vi "Thermistor_Callibration.vi"(11 "DataCluster in":T2={"Core"={"Current VI Reference"=refnum, "Close Panel on Exit?"=FALSE, "Exit"=FALSE, "Initialized?"=FALSE}, "Connections"={"cDAQ"={"Task"="", "Connected"=FALSE, "Active"=FALSE, "ID"=""}, "Camera"={"Session"="", "Connected"=FALSE, "Active"=FALSE, "Placeholder"=refnum}, "PSU"={"Port"="", "Connected"=FALSE, "Active"=FALSE}, "Arduino"={"Port"="", "Connected"=FALSE, "Active"=FALSE}}, "Data Acquisition"={"Setup"={"Label"="", "Operator"="", "Notes"="", "TempGrad"=1.0, "TargetTemp"=1.0, "Sample Volume"=1.0}, "Camera"={"Image"=refnum, "Save Image"=refnum, "Image Frequency"=20, "Rectangle"={"Left"=0, "Top"=0, "Right"=0, "Bottom"=0, "Rotation"=0.0}, "Calibration"={"Top Left"={"X"=0.0, "Y"=0.0}, "Top Right"={"X"=0.0, "Y"=0.0}, "Bottom Left"={"X"=0.0, "Y"=0.0}, "Bottom Right"={"X"=0.0, "Y"=0.0}, "Fixpoint"={"X"=0.0, "Y"=0.0}, "Scan Area"=0.0, "Fixpoint Area"=0.0, "Well Pixels"=[], "Valid"=FALSE}, "FocusPos"=0, "Display Mapping"=10}, "Thermistor"={"Sample Size"=1, "Calibration"={"B0.100"=[], "R25"=[], "c"=[], "State"=[], "V_S"=5.0, "R_S"=100.0}, "Timing Mode"=14713}, "Partition"={"Data"=[], "Cell Label"="", "Cell Color"=0, "Height"=10, "Width"=16, "Grid"=[]}, "Queue"={"Size"=1, "Queue"=refnum}, "Sample Rate"=1, "Active"=FALSE, "Ready"=FALSE, "Graph Mode"=0}, "Control"={"Sample Rate"=1, "PID gains"={"proportional gain (Kc)"=1.0, "integral time (Ti, min)"=0.01, "derivative time (Td, min)"=0.0}}} {"Control"."PID gains"."derivative time (Td, min)" format="%.3f"; "Control"."PID gains"."integral time (Ti, min)" format="%.3f"; "Control"."PID gains"."proportional gain (Kc)" format="%.3f"; "Control"."Sample Rate" min=1 max=20 step=1 format="%.0f Samples/sec"; "Data Acquisition"."Graph Mode" items=["Thermistor Temperature", "Camera Temperature"]; "Data Acquisition"."Thermistor"."Timing Mode" items=["Automatic"=16097, "High Resolution"=10195, "High Speed"=14712, "Best 50 Hz Rejection"=14713, "Best 60 Hz Rejection"=14714, "Custom"=10137]; "Data Acquisition"."Thermistor"."Calibration"."R_S" min=0.1 max=1000.0 format="%#_g kOhm"; "Data Acquisition"."Thermistor"."Calibration"."V_S" min=5.0 max=48.0 format="%#_g V"; "Data Acquisition"."Thermistor"."Calibration"."R25" min=0.1 max=1000.0 format="%#_g kOhm"; "Data Acquisition"."Thermistor"."Calibration"."B0.100" min=100.0 max=10000.0 format="%#_g K"; "Data Acquisition"."Thermistor"."Sample Size" min=1 max=200; "Data Acquisition"."Sample Rate" min=20 max=240 format="%.0f samples/min"; "Data Acquisition"."Queue"."Size" min=1 max=200; "Data Acquisition"."Camera"."Display Mapping" items=["Default"=10, "Most Significant Bits"=11, "Full Dynamic"=12, "Downshift"=13, "Given Range"=14, "90% Dynamic"=15, "Given Percent Range"=16]; "Data Acquisition"."Camera"."Calibration"."Fixpoint"."Y" format="%.2f"; "Data Acquisition"."Camera"."Calibration"."Fixpoint"."X" format="%.2f"; "Data Acquisition"."Camera"."Calibration"."Top Left"."Y" format="%.2f"; "Data Acquisition"."Camera"."Calibration"."Top Left"."X" format="%.2f"; "Data Acquisition"."Camera"."Calibration"."Top Right"."Y" format="%.2f"; "Data Acquisition"."Camera"."Calibration"."Top Right"."X" format="%.2f"; "Data Acquisition"."Camera"."Calibration"."Bottom Left"."Y" format="%.2f"; "Data Acquisition"."Camera"."Calibration"."Bottom Left"."X" format="%.2f"; "Data Acquisition"."Camera"."Calibration"."Bottom Right"."Y" format="%.2f"; "Data Acquisition"."Camera"."Calibration"."Bottom Right"."X" format="%.2f"; "Data Acquisition"."Camera"."Rectangle"."Rotation" min=-90.0 max=90.0 step=1.0 format="%.2f"; "Data Acquisition"."Camera"."Rectangle"."Left" scale=0.0..1024.0; "Data Acquisition"."Camera"."Rectangle"."Right" scale=0.0..1024.0; "Data Acquisition"."Camera"."Image Frequency" min=1 max=60 step=1; "Data Acquisition"."Setup"."Sample Volume" min=0.0 max=500.0 format="%#_g µL"; "Data Acquisition"."Setup"."TargetTemp" min=-40.0 max=40.0 step=0.5 format="%#_g °C"; "Data Acquisition"."Setup"."TempGrad" min=-100.0 max=100.0 step=0.1 format="%#_g °C/min"}) -> (2 "State Out":string="Data: Save Calibration", 3 "DataCluster out":T2={"Core"={"Current VI Reference"=refnum, "Close Panel on Exit?"=FALSE, "Exit"=FALSE, "Initialized?"=FALSE}, "Connections"={"cDAQ"={"Task"="", "Connected"=FALSE, "Active"=FALSE, "ID"=""}, "Camera"={"Session"="", "Connected"=FALSE, "Active"=FALSE, "Placeholder"=refnum}, "PSU"={"Port"="", "Connected"=FALSE, "Active"=FALSE}, "Arduino"={"Port"="", "Connected"=FALSE, "Active"=FALSE}}, "Data Acquisition"={"Setup"={"Label"="", "Operator"="", "Notes"="", "TempGrad"=0.0, "TargetTemp"=0.0, "Sample Volume"=0.0}, "Camera"={"Image"=refnum, "Save Image"=refnum, "Image Frequency"=20, "Rectangle"={"Left"=0, "Top"=0, "Right"=0, "Bottom"=0, "Rotation"=0.0}, "Calibration"={"Top Left"={"X"=0.0, "Y"=0.0}, "Top Right"={"X"=0.0, "Y"=0.0}, "Bottom Left"={"X"=0.0, "Y"=0.0}, "Bottom Right"={"X"=0.0, "Y"=0.0}, "Fixpoint"={"X"=0.0, "Y"=0.0}, "Scan Area"=0.0, "Fixpoint Area"=0.0, "Well Pixels"=[], "Valid"=FALSE}, "FocusPos"=0, "Display Mapping"=10}, "Thermistor"={"Sample Size"=0, "Calibration"={"B0.100"=[], "R25"=[], "c"=[], "State"=[], "V_S"=0.0, "R_S"=0.0}, "Timing Mode"=0}, "Partition"={"Data"=[], "Cell Label"="", "Cell Color"=0, "Height"=0, "Width"=0, "Grid"=[]}, "Queue"={"Size"=0, "Queue"=refnum}, "Sample Rate"=0, "Active"=FALSE, "Ready"=FALSE, "Graph Mode"=0}, "Control"={"Sample Rate"=0, "PID gains"={"proportional gain (Kc)"=0.0, "integral time (Ti, min)"=0.0, "derivative time (Td, min)"=0.0}}} {"Control"."PID gains"."derivative time (Td, min)" format="%.3f"; "Control"."PID gains"."integral time (Ti, min)" format="%.3f"; "Control"."PID gains"."proportional gain (Kc)" format="%.3f"; "Control"."Sample Rate" min=1 max=20 step=1 format="%.0f Samples/sec"; "Data Acquisition"."Graph Mode" items=["Thermistor Temperature", "Camera Temperature"]; "Data Acquisition"."Thermistor"."Timing Mode" items=["Automatic"=16097, "High Resolution"=10195, "High Speed"=14712, "Best 50 Hz Rejection"=14713, "Best 60 Hz Rejection"=14714, "Custom"=10137]; "Data Acquisition"."Thermistor"."Calibration"."R_S" min=0.1 max=1000.0 format="%#_g kOhm"; "Data Acquisition"."Thermistor"."Calibration"."V_S" min=5.0 max=48.0 format="%#_g V"; "Data Acquisition"."Thermistor"."Calibration"."R25" min=0.1 max=1000.0 format="%#_g kOhm"; "Data Acquisition"."Thermistor"."Calibration"."B0.100" min=100.0 max=10000.0 format="%#_g K"; "Data Acquisition"."Thermistor"."Sample Size" min=1 max=200; "Data Acquisition"."Sample Rate" min=20 max=240 format="%.0f samples/min"; "Data Acquisition"."Queue"."Size" min=1 max=200; "Data Acquisition"."Camera"."Display Mapping" items=["Default"=10, "Most Significant Bits"=11, "Full Dynamic"=12, "Downshift"=13, "Given Range"=14, "90% Dynamic"=15, "Given Percent Range"=16]; "Data Acquisition"."Camera"."Calibration"."Fixpoint"."Y" format="%.2f"; "Data Acquisition"."Camera"."Calibration"."Fixpoint"."X" format="%.2f"; "Data Acquisition"."Camera"."Calibration"."Top Left"."Y" format="%.2f"; "Data Acquisition"."Camera"."Calibration"."Top Left"."X" format="%.2f"; "Data Acquisition"."Camera"."Calibration"."Top Right"."Y" format="%.2f"; "Data Acquisition"."Camera"."Calibration"."Top Right"."X" format="%.2f"; "Data Acquisition"."Camera"."Calibration"."Bottom Left"."Y" format="%.2f"; "Data Acquisition"."Camera"."Calibration"."Bottom Left"."X" format="%.2f"; "Data Acquisition"."Camera"."Calibration"."Bottom Right"."Y" format="%.2f"; "Data Acquisition"."Camera"."Calibration"."Bottom Right"."X" format="%.2f"; "Data Acquisition"."Camera"."Rectangle"."Rotation" min=-90.0 max=90.0 step=1.0 format="%.2f"; "Data Acquisition"."Camera"."Rectangle"."Left" scale=0.0..1024.0; "Data Acquisition"."Camera"."Rectangle"."Right" scale=0.0..1024.0; "Data Acquisition"."Camera"."Image Frequency" min=1 max=60 step=1; "Data Acquisition"."Setup"."Sample Volume" min=0.0 max=500.0 format="%#_g µL"; "Data Acquisition"."Setup"."TargetTemp" min=-40.0 max=40.0 step=0.5 format="%#_g °C"; "Data Acquisition"."Setup"."TempGrad" min=-100.0 max=100.0 step=0.1 format="%#_g °C/min"})   [LabVIEW 2020]
uses:
  DataCluster.ctl
  <vilib>/userDefined/High Color/IMAQdx.ctl
  <vilib>/vision/Image Controls.llb/IMAQ Image.ctl
panel:
  in  "Ring":u16(ring) items=["Setup", "Thermistor 1", "Thermistor 2", "Thermistor 3", "Thermistor 4", "Thermistor 5", "Thermistor 6", "Thermistor 7", "Thermistor 8"]
  out "Tab Control":T1(tab)
  in  "Supply Voltage":dbl=12.062 format="%#_g V"
  in  "Static Resistor":dbl=10.0 min=0.1 max=1000.0 format="%#_g kOhm"
  in  "Active":bool
  in  "c":dbl[](array[numeric]) caption="constants" format="%_6g"
  in  "B0.100":dbl caption="ß0.100" min=0.0 format="%#_g K"
  in  "R25":dbl min=0.0 format="%#_g kOhm"
  in  "Active 2":bool
  in  "B0.100 2":dbl caption="ß0.100" min=0.0 format="%#_g K"
  in  "R25 2":dbl caption="R25" min=0.0 format="%#_g kOhm"
  in  "c 2":dbl[](array[numeric]) caption="constants" format="%_6g"
  in  "Active 3":bool
  in  "B0.100 3":dbl caption="ß0.100" min=0.0 format="%#_g K"
  in  "R25 3":dbl caption="R25" min=0.0 format="%#_g kOhm"
  in  "c 3":dbl[](array[numeric]) caption="constants" format="%_6g"
  in  "Active 4":bool
  in  "B0.100 4":dbl caption="ß0.100" min=0.0 format="%#_g K"
  in  "R25 4":dbl caption="R25" min=0.0 format="%#_g kOhm"
  in  "c 4":dbl[](array[numeric]) caption="constants" format="%_6g"
  in  "Active 5":bool
  in  "B0.100 5":dbl caption="ß0.100" min=0.0 format="%#_g K"
  in  "R25 5":dbl caption="R25" min=0.0 format="%#_g kOhm"
  in  "c 5":dbl[](array[numeric]) caption="constants" format="%_6g"
  in  "Active 6":bool
  in  "B0.100 6":dbl caption="ß0.100" min=0.0 format="%#_g K"
  in  "R25 6":dbl caption="R25" min=0.0 format="%#_g kOhm"
  in  "c 6":dbl[](array[numeric]) caption="constants" format="%_6g"
  in  "Active 7":bool
  in  "B0.100 7":dbl caption="ß0.100" min=0.0 format="%#_g K"
  in  "R25 7":dbl caption="R25" min=0.0 format="%#_g kOhm"
  in  "c 7":dbl[](array[numeric]) caption="constants" format="%_6g"
  in  "Active 8":bool
  in  "B0.100 8":dbl caption="ß0.100" min=0.0 format="%#_g K"
  in  "R25 8":dbl caption="R25" min=0.0 format="%#_g kOhm"
  in  "c 8":dbl[](array[numeric]) caption="constants" format="%_6g"
  in  "Cancel":bool
  in  "OK":bool
  # "Adjust thermistor calibration values used in conversion between measured voltages and temperatures"
  # "c0"
  # "c1"
  # "c2"
  # "c3"
  # "c4"
  # "c0"
  # "c1"
  # "c2"
  # "c3"
  # "c4"
  # "c0"
  # "c1"
  # "c2"
  # "c3"
  # "c4"
  # "c0"
  # "c1"
  # "c2"
  # "c3"
  # "c4"
  # "c0"
  # "c1"
  # "c2"
  # "c3"
  # "c4"
  # "c0"
  # "c1"
  # "c2"
  # "c3"
  # "c4"
  # "c0"
  # "c1"
  # "c2"
  # "c3"
  # "c4"
  # "c0"
  # "c1"
  # "c2"
  # "c3"
  # "c4"
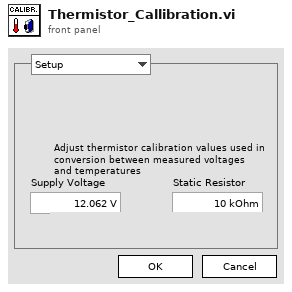
[diagram p1: front panel]
types:
  T1 = enum32{"Setup", "1", "2", "3", "4", "5", "6", "7", "8"}
  T2 = typedef "DataCluster.ctl" = cluster{"Core":cluster{"Current VI Reference":refnum<vi>, "Close Panel on Exit?":bool, "Exit":bool, "Initialized?":bool}, "Connections":cluster{"cDAQ":cluster{"Task":refnum<k21>, "Connected":bool, "Active":bool, "ID":string}, "Camera":cluster{"Session":T3, "Connected":bool, "Active":bool, "Placeholder":T4}, "PSU":cluster{"Port":refnum<visa-resource-name>, "Connected":bool, "Active":bool}, "Arduino":cluster{"Port":refnum<visa-resource-name>, "Connected":bool, "Active":bool}}, "Data Acquisition":cluster{"Setup":cluster{"Label":string, "Operator":string, "Notes":string, "TempGrad":dbl, "TargetTemp":dbl, "Sample Volume":dbl}, "Camera":cluster{"Image":T4, "Save Image":T4, "Image Frequency":i32, "Rectangle":T5, "Calibration":cluster{"Top Left":T6, "Top Right":T6, "Bottom Left":T6, "Bottom Right":T6, "Fixpoint":T6, "Scan Area":dbl, "Fixpoint Area":dbl, "Well Pixels":cluster{"X":i32, "Y":i32}[][], "Valid":bool}, "FocusPos":u32, "Display Mapping":u32}, "Thermistor":cluster{"Sample Size":i32, "Calibration":cluster{"B0.100":dbl[], "R25":dbl[], "c":dbl[][], "State":bool[], "V_S":dbl, "R_S":dbl}, "Timing Mode":i32}, "Partition":cluster{"Data":string[][], "Cell Label":string, "Cell Color":u32, "Height":i32, "Width":i32, "Grid":string[][]}, "Queue":cluster{"Size":i32, "Queue":refnum<queue>}, "Sample Rate":i32, "Active":bool, "Ready":bool, "Graph Mode":u16}, "Control":cluster{"Sample Rate":i32, "PID gains":cluster{"proportional gain (Kc)":dbl, "integral time (Ti, min)":dbl, "derivative time (Td, min)":dbl}}}
  T3 = typedef "IMAQdx.ctl" = refnum<k21>
  T4 = typedef "IMAQ Image.ctl" = refnum<image>
  T5 = typedef "IMAQ Rectangle" = cluster{"Left":i32, "Top":i32, "Right":i32, "Bottom":i32, "Rotation":dbl}
  T6 = typedef "IMAQ Point" = cluster{"X":sgl, "Y":sgl}
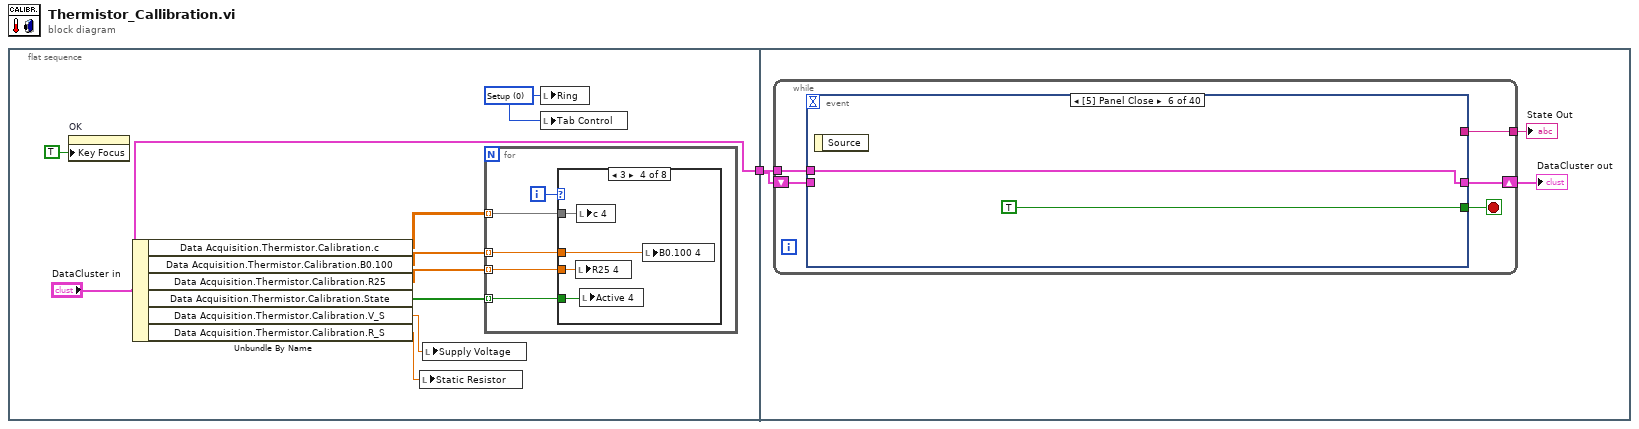
[diagram p0: block diagram]
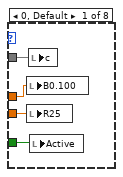
[diagram p2: hidden frame]
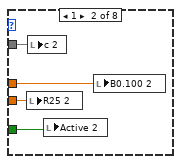
[diagram p3: hidden frame]
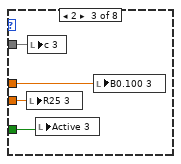
[diagram p4: hidden frame]
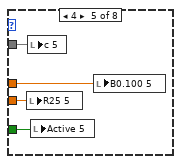
[diagram p5: hidden frame]
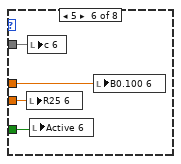
[diagram p6: hidden frame]
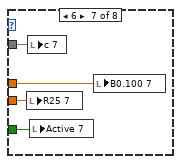
[diagram p7: hidden frame]
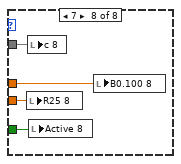
[diagram p8: hidden frame]
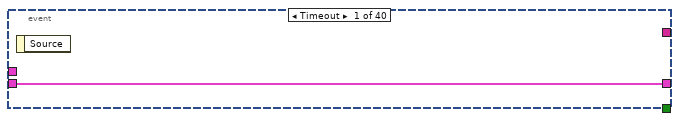
[diagram p9: hidden frame]
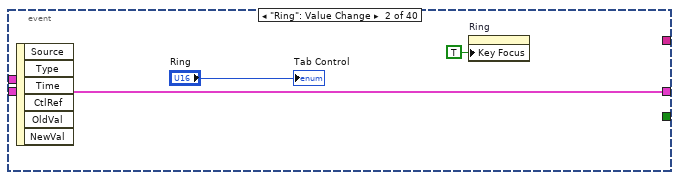
[diagram p10: hidden frame]
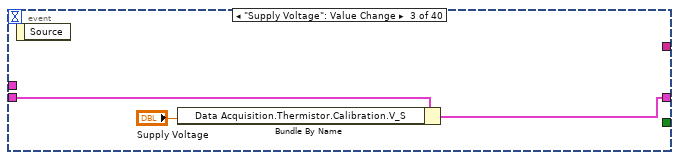
[diagram p11: hidden frame]
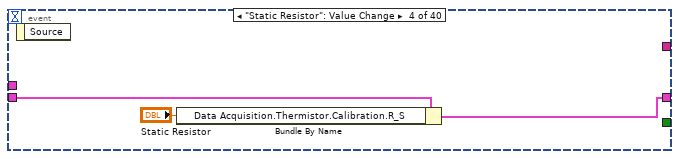
[diagram p12: hidden frame]
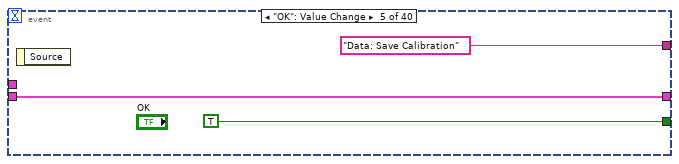
[diagram p13: hidden frame]
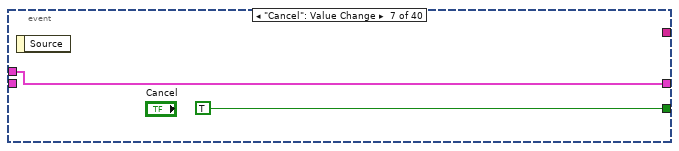
[diagram p14: hidden frame]
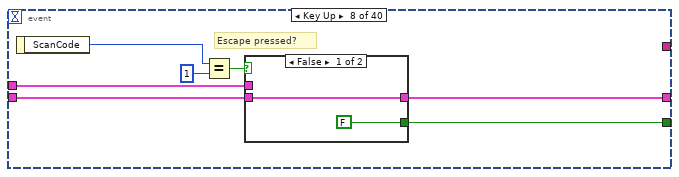
[diagram p15: hidden frame]
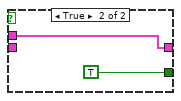
[diagram p16: hidden frame]
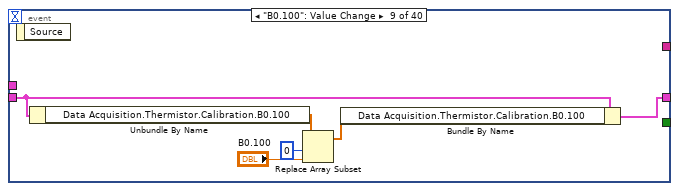
[diagram p17: hidden frame]
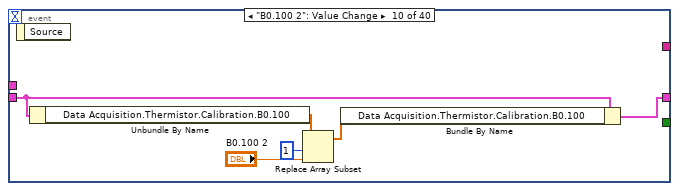
[diagram p18: hidden frame]
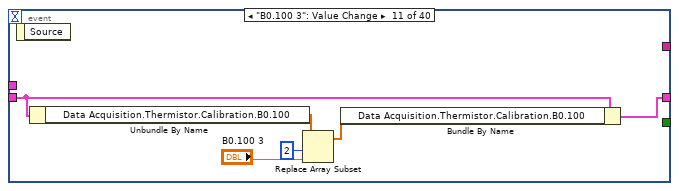
[diagram p19: hidden frame]
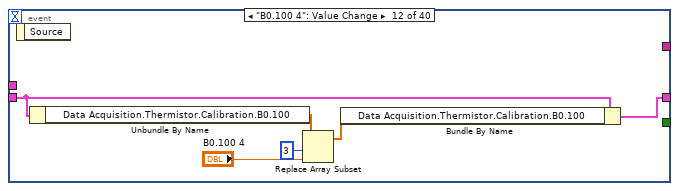
[diagram p20: hidden frame]
diagram:
  n1 = flat-sequence {
    tunnel: ["DataCluster in"] -> w1
    tunnel: w1 -> [w50]
    frame #0 {
      w4 = u16 0 items=["Setup", "Thermistor 1", "Thermistor 2", "Thermistor 3", "Thermistor 4", "Thermistor 5", "Thermistor 6", "Thermistor 7", "Thermistor 8"] ("Ring")
      n2 = property on="OK" class="Bool"("Key Focus"=TRUE) -> ()  [unwired: 2 in, 2 out]
      n3 = Unbundle By Name("DataCluster in") -> ("Data Acquisition.Thermistor.Calibration.c"=w3:dbl[][], "Data Acquisition.Thermistor.Calibration.B0.100"=w5:dbl[], "Data Acquisition.Thermistor.Calibration.R25"=w6:dbl[], "Data Acquisition.Thermistor.Calibration.State"=w2:bool[], "Data Acquisition.Thermistor.Calibration.V_S"=w8:dbl, "Data Acquisition.Thermistor.Calibration.R_S"=w7:dbl)
      n4 = local write "Static Resistor"(w7) -> ()
      n5 = local write "Supply Voltage"(w8) -> ()
      n6 = for {
        tunnel: w6 -> [w14] mode=indexing
        tunnel: w5 -> [w13] mode=indexing
        tunnel: w3 -> [w12] mode=indexing
        tunnel: w2 -> [w11] mode=indexing
        i -> [w15]
        n7 = case shown="3" w15 {
          tunnel: w14 -> [w19 w23 w27 w31 w35 w39 w43 w47]
          tunnel: w13 -> [w18 w22 w26 w30 w34 w38 w42 w46]
          tunnel: w12 -> [w17 w21 w25 w29 w33 w37 w41 w45]
          tunnel: w11 -> [w16 w20 w24 w28 w32 w36 w40 w44]
          frame 0, Default {
            n8 = local write "B0.100"(w18) -> ()
            n9 = local write "R25"(w19) -> ()
            n10 = local write "c"(w17) -> ()
            n11 = local write "Active"(w16) -> ()
          }
          frame 1 {
            n12 = local write "R25 2"(w23) -> ()
            n13 = local write "c 2"(w21) -> ()
            n14 = local write "Active 2"(w20) -> ()
            n15 = local write "B0.100 2"(w22) -> ()
          }
          frame 2 {
            n16 = local write "R25 3"(w27) -> ()
            n17 = local write "c 3"(w25) -> ()
            n18 = local write "Active 3"(w24) -> ()
            n19 = local write "B0.100 3"(w26) -> ()
          }
          frame 3 {
            n20 = local write "R25 4"(w31) -> ()
            n21 = local write "c 4"(w29) -> ()
            n22 = local write "Active 4"(w28) -> ()
            n23 = local write "B0.100 4"(w30) -> ()
          }
          frame 4 {
            n24 = local write "R25 5"(w35) -> ()
            n25 = local write "c 5"(w33) -> ()
            n26 = local write "Active 5"(w32) -> ()
            n27 = local write "B0.100 5"(w34) -> ()
          }
          frame 5 {
            n28 = local write "R25 6"(w39) -> ()
            n29 = local write "c 6"(w37) -> ()
            n30 = local write "Active 6"(w36) -> ()
            n31 = local write "B0.100 6"(w38) -> ()
          }
          frame 6 {
            n32 = local write "R25 7"(w43) -> ()
            n33 = local write "c 7"(w41) -> ()
            n34 = local write "Active 7"(w40) -> ()
            n35 = local write "B0.100 7"(w42) -> ()
          }
          frame 7 {
            n36 = local write "R25 8"(w47) -> ()
            n37 = local write "c 8"(w45) -> ()
            n38 = local write "Active 8"(w44) -> ()
            n39 = local write "B0.100 8"(w46) -> ()
          }
        }
      }
      n40 = local write "Ring"(w4) -> ()
      n41 = local write "Tab Control"(w4) -> ()
    }
    frame #1 {
      n42 = while {
        shift-right: [w55] -> w49
        shift-left: w50 -> [w54]
        tunnel: w50 -> [w53]
        tunnel: [w51] -> w48
        stop <- w52 stop-if-true
        n43 = event shown="[5] Panel Close" {
          selector: _ -> [_ _ _ _ _ _ _ _ _ _ _ _ _ _ _ _ _ _ _ _ _ _ _ _ _ _ _ _ _ _ _ _ _ _ _ _ _ _ _ _]
          dyn-events: _ -> [_ _ _ _ _ _ _ _ _ _ _ _ _ _ _ _ _ _ _ _ _ _ _ _ _ _ _ _ _ _ _ _ _ _ _ _ _ _ _ _]
          timeout: _ -> [_ _ _ _ _ _ _ _ _ _ _ _ _ _ _ _ _ _ _ _ _ _ _ _ _ _ _ _ _ _ _ _ _ _ _ _ _ _ _ _]
          tunnel: w54 -> [w56 w58 w62 w65 w68 _ _ w73 w88 w94 w100 w106 w112 w118 w124 w130 w136 w142 w148 w154 w160 w166 w172 w178 w184 w190 w196 w202 w208 w214 w220 w226 w232 w238 w244 w250 w256 w262 w268 w274]
          tunnel: [w56 w58 w61 w64 w68 w69 w72 w75 w89 w95 w101 w107 w113 w119 w125 w131 w137 w143 w149 w155 w161 w167 w173 w179 w185 w191 w197 w203 w209 w215 w221 w227 w233 w239 w245 w251 w257 w263 w269 w275] -> w55
          tunnel: w53 -> [_ _ _ _ _ w69 w72 w74 _ _ _ _ _ _ _ _ _ _ _ _ _ _ _ _ _ _ _ _ _ _ _ _ _ _ _ _ _ _ _ _]
          tunnel: [_ _ _ _ TRUE TRUE TRUE w79 _ _ _ _ _ _ _ _ _ _ _ _ _ _ _ _ _ _ _ _ _ _ _ _ _ _ _ _ _ _ _ _] -> w52
          tunnel: [_ _ _ _ "Data: Save Calibration" _ _ _ _ _ _ _ _ _ _ _ _ _ _ _ _ _ _ _ _ _ _ _ _ _ _ _ _ _ _ _ _ _ _ _] -> w51
          event Timeout {
            n44 = event-data() -> ()  [unwired: 1 in, 1 out]
          }
          event "Ring": Value Change {
            n45 = event-data() -> ()  [unwired: 1 in, 6 out]
            n46 = property on="Ring" class="Ring (strict)"("Key Focus"=TRUE) -> ()  [unwired: 2 in, 2 out]
            "Tab Control" <- "Ring"
          }
          event "Supply Voltage": Value Change {
            n47 = event-data() -> ()  [unwired: 1 in, 1 out]
            n48 = Bundle By Name(cluster=w62, "Data Acquisition.Thermistor.Calibration.V_S"="Supply Voltage") -> (w61:T2)
          }
          event "Static Resistor": Value Change {
            n49 = event-data() -> ()  [unwired: 1 in, 1 out]
            n50 = Bundle By Name(cluster=w65, "Data Acquisition.Thermistor.Calibration.R_S"="Static Resistor") -> (w64:T2)
          }
          event "OK": Value Change {
            n51 = event-data() -> ()  [unwired: 1 in, 1 out]
          }
          event Panel Close {
            n52 = event-data() -> ()  [unwired: 1 in, 1 out]
          }
          event "Cancel": Value Change {
            n53 = event-data() -> ()  [unwired: 1 in, 1 out]
          }
          event Key Up {
            # "Escape pressed?"
            n54 = event-data() -> ("ScanCode"=w78:i16)  [unwired: 1 in]
            n55 = Equal?(x=w78, y=i16 1) -> (x = y?=w76:bool)
            n56 = case shown="False" w76 {
              tunnel: [FALSE TRUE] -> w79
              tunnel: [w81 w82] -> w75
              tunnel: w74 -> [_ w82]
              tunnel: w73 -> [w81 _]
              frame False {
              }
              frame True {
              }
            }
          }
          event "B0.100": Value Change {
            n57 = event-data() -> ()  [unwired: 1 in, 1 out]
            n58 = Unbundle By Name(w88) -> ("Data Acquisition.Thermistor.Calibration.B0.100"=w87:dbl[])
            n59 = Replace Array Subset(array=w87, new element="B0.100", index=0) -> (w84:dbl[])
            n60 = Bundle By Name(cluster=w88, "Data Acquisition.Thermistor.Calibration.B0.100"=w84) -> (w89:T2)
          }
          event "B0.100 2": Value Change {
            n61 = event-data() -> ()  [unwired: 1 in, 1 out]
            n62 = Unbundle By Name(w94) -> ("Data Acquisition.Thermistor.Calibration.B0.100"=w93:dbl[])
            n63 = Replace Array Subset(array=w93, new element="B0.100 2", index=1) -> (w91:dbl[])
            n64 = Bundle By Name(cluster=w94, "Data Acquisition.Thermistor.Calibration.B0.100"=w91) -> (w95:T2)
          }
          event "B0.100 3": Value Change {
            n65 = event-data() -> ()  [unwired: 1 in, 1 out]
            n66 = Unbundle By Name(w100) -> ("Data Acquisition.Thermistor.Calibration.B0.100"=w99:dbl[])
            n67 = Replace Array Subset(array=w99, new element="B0.100 3", index=2) -> (w97:dbl[])
            n68 = Bundle By Name(cluster=w100, "Data Acquisition.Thermistor.Calibration.B0.100"=w97) -> (w101:T2)
          }
          event "B0.100 4": Value Change {
            n69 = event-data() -> ()  [unwired: 1 in, 1 out]
            n70 = Unbundle By Name(w106) -> ("Data Acquisition.Thermistor.Calibration.B0.100"=w105:dbl[])
            n71 = Replace Array Subset(array=w105, new element="B0.100 4", index=3) -> (w103:dbl[])
            n72 = Bundle By Name(cluster=w106, "Data Acquisition.Thermistor.Calibration.B0.100"=w103) -> (w107:T2)
          }
          event "B0.100 5": Value Change {
            n73 = event-data() -> ()  [unwired: 1 in, 1 out]
            n74 = Unbundle By Name(w112) -> ("Data Acquisition.Thermistor.Calibration.B0.100"=w111:dbl[])
            n75 = Replace Array Subset(array=w111, new element="B0.100 5", index=4) -> (w109:dbl[])
            n76 = Bundle By Name(cluster=w112, "Data Acquisition.Thermistor.Calibration.B0.100"=w109) -> (w113:T2)
          }
          event "B0.100 6": Value Change {
            n77 = event-data() -> ()  [unwired: 1 in, 1 out]
            n78 = Unbundle By Name(w118) -> ("Data Acquisition.Thermistor.Calibration.B0.100"=w117:dbl[])
            n79 = Replace Array Subset(array=w117, new element="B0.100 6", index=5) -> (w115:dbl[])
            n80 = Bundle By Name(cluster=w118, "Data Acquisition.Thermistor.Calibration.B0.100"=w115) -> (w119:T2)
          }
          event "B0.100 7": Value Change {
            n81 = event-data() -> ()  [unwired: 1 in, 1 out]
            n82 = Unbundle By Name(w124) -> ("Data Acquisition.Thermistor.Calibration.B0.100"=w123:dbl[])
            n83 = Replace Array Subset(array=w123, new element="B0.100 7", index=6) -> (w121:dbl[])
            n84 = Bundle By Name(cluster=w124, "Data Acquisition.Thermistor.Calibration.B0.100"=w121) -> (w125:T2)
          }
          event "B0.100 8": Value Change {
            n85 = event-data() -> ()  [unwired: 1 in, 1 out]
            n86 = Unbundle By Name(w130) -> ("Data Acquisition.Thermistor.Calibration.B0.100"=w129:dbl[])
            n87 = Replace Array Subset(array=w129, new element="B0.100 8", index=7) -> (w127:dbl[])
            n88 = Bundle By Name(cluster=w130, "Data Acquisition.Thermistor.Calibration.B0.100"=w127) -> (w131:T2)
          }
          event "R25": Value Change {
            n89 = event-data() -> ()  [unwired: 1 in, 1 out]
            n90 = Unbundle By Name(w136) -> ("Data Acquisition.Thermistor.Calibration.R25"=w135:dbl[])
            n91 = Replace Array Subset(array=w135, new element="R25", index=0) -> (w133:dbl[])
            n92 = Bundle By Name(cluster=w136, "Data Acquisition.Thermistor.Calibration.R25"=w133) -> (w137:T2)
          }
          event "R25 2": Value Change {
            n93 = event-data() -> ()  [unwired: 1 in, 1 out]
            n94 = Unbundle By Name(w142) -> ("Data Acquisition.Thermistor.Calibration.R25"=w141:dbl[])
            n95 = Replace Array Subset(array=w141, new element="R25 2", index=1) -> (w139:dbl[])
            n96 = Bundle By Name(cluster=w142, "Data Acquisition.Thermistor.Calibration.R25"=w139) -> (w143:T2)
          }
          event "R25 3": Value Change {
            n97 = event-data() -> ()  [unwired: 1 in, 1 out]
            n98 = Unbundle By Name(w148) -> ("Data Acquisition.Thermistor.Calibration.R25"=w147:dbl[])
            n99 = Replace Array Subset(array=w147, new element="R25 3", index=2) -> (w145:dbl[])
            n100 = Bundle By Name(cluster=w148, "Data Acquisition.Thermistor.Calibration.R25"=w145) -> (w149:T2)
          }
          event "R25 4": Value Change {
            n101 = event-data() -> ()  [unwired: 1 in, 1 out]
            n102 = Unbundle By Name(w154) -> ("Data Acquisition.Thermistor.Calibration.R25"=w153:dbl[])
            n103 = Replace Array Subset(array=w153, new element="R25 4", index=3) -> (w151:dbl[])
            n104 = Bundle By Name(cluster=w154, "Data Acquisition.Thermistor.Calibration.R25"=w151) -> (w155:T2)
          }
          event "R25 5": Value Change {
            n105 = event-data() -> ()  [unwired: 1 in, 1 out]
            n106 = Unbundle By Name(w160) -> ("Data Acquisition.Thermistor.Calibration.R25"=w159:dbl[])
            n107 = Replace Array Subset(array=w159, new element="R25 5", index=4) -> (w157:dbl[])
            n108 = Bundle By Name(cluster=w160, "Data Acquisition.Thermistor.Calibration.R25"=w157) -> (w161:T2)
          }
          event "R25 6": Value Change {
            n109 = event-data() -> ()  [unwired: 1 in, 1 out]
            n110 = Unbundle By Name(w166) -> ("Data Acquisition.Thermistor.Calibration.R25"=w165:dbl[])
            n111 = Replace Array Subset(array=w165, new element="R25 6", index=5) -> (w163:dbl[])
            n112 = Bundle By Name(cluster=w166, "Data Acquisition.Thermistor.Calibration.R25"=w163) -> (w167:T2)
          }
          event "R25 7": Value Change {
            n113 = event-data() -> ()  [unwired: 1 in, 1 out]
            n114 = Unbundle By Name(w172) -> ("Data Acquisition.Thermistor.Calibration.R25"=w171:dbl[])
            n115 = Replace Array Subset(array=w171, new element="R25 7", index=6) -> (w169:dbl[])
            n116 = Bundle By Name(cluster=w172, "Data Acquisition.Thermistor.Calibration.R25"=w169) -> (w173:T2)
          }
          event "R25 8": Value Change {
            n117 = event-data() -> ()  [unwired: 1 in, 1 out]
            n118 = Unbundle By Name(w178) -> ("Data Acquisition.Thermistor.Calibration.R25"=w177:dbl[])
            n119 = Replace Array Subset(array=w177, new element="R25 8", index=7) -> (w175:dbl[])
            n120 = Bundle By Name(cluster=w178, "Data Acquisition.Thermistor.Calibration.R25"=w175) -> (w179:T2)
          }
          event "c": Value Change {
            n121 = event-data() -> ()  [unwired: 1 in, 1 out]
            n122 = Unbundle By Name(w184) -> ("Data Acquisition.Thermistor.Calibration.c"=w183:dbl[][])
            n123 = Replace Array Subset(array=w183, new element="c", index (row)=0 ("index")) -> (w181:dbl[][])  [unwired: 1 in]
            n124 = Bundle By Name(cluster=w184, "Data Acquisition.Thermistor.Calibration.c"=w181) -> (w185:T2)
          }
          event "c 2": Value Change {
            n125 = event-data() -> ()  [unwired: 1 in, 1 out]
            n126 = Unbundle By Name(w190) -> ("Data Acquisition.Thermistor.Calibration.c"=w189:dbl[][])
            n127 = Replace Array Subset(array=w189, new element="c 2", index (row)=1 ("index")) -> (w187:dbl[][])  [unwired: 1 in]
            n128 = Bundle By Name(cluster=w190, "Data Acquisition.Thermistor.Calibration.c"=w187) -> (w191:T2)
          }
          event "c 3": Value Change {
            n129 = event-data() -> ()  [unwired: 1 in, 1 out]
            n130 = Unbundle By Name(w196) -> ("Data Acquisition.Thermistor.Calibration.c"=w195:dbl[][])
            n131 = Replace Array Subset(array=w195, new element="c 3", index (row)=2 ("index")) -> (w193:dbl[][])  [unwired: 1 in]
            n132 = Bundle By Name(cluster=w196, "Data Acquisition.Thermistor.Calibration.c"=w193) -> (w197:T2)
          }
          event "c 4": Value Change {
            n133 = event-data() -> ()  [unwired: 1 in, 1 out]
            n134 = Unbundle By Name(w202) -> ("Data Acquisition.Thermistor.Calibration.c"=w201:dbl[][])
            n135 = Replace Array Subset(array=w201, new element="c 4", index (row)=3 ("index")) -> (w199:dbl[][])  [unwired: 1 in]
            n136 = Bundle By Name(cluster=w202, "Data Acquisition.Thermistor.Calibration.c"=w199) -> (w203:T2)
          }
          event "c 5": Value Change {
            n137 = event-data() -> ()  [unwired: 1 in, 1 out]
            n138 = Unbundle By Name(w208) -> ("Data Acquisition.Thermistor.Calibration.c"=w207:dbl[][])
            n139 = Replace Array Subset(array=w207, new element="c 5", index (row)=4 ("index")) -> (w205:dbl[][])  [unwired: 1 in]
            n140 = Bundle By Name(cluster=w208, "Data Acquisition.Thermistor.Calibration.c"=w205) -> (w209:T2)
          }
          event "c 6": Value Change {
            n141 = event-data() -> ()  [unwired: 1 in, 1 out]
            n142 = Unbundle By Name(w214) -> ("Data Acquisition.Thermistor.Calibration.c"=w213:dbl[][])
            n143 = Replace Array Subset(array=w213, new element="c 6", index (row)=5 ("index")) -> (w211:dbl[][])  [unwired: 1 in]
            n144 = Bundle By Name(cluster=w214, "Data Acquisition.Thermistor.Calibration.c"=w211) -> (w215:T2)
          }
          event "c 7": Value Change {
            n145 = event-data() -> ()  [unwired: 1 in, 1 out]
            n146 = Unbundle By Name(w220) -> ("Data Acquisition.Thermistor.Calibration.c"=w219:dbl[][])
            n147 = Replace Array Subset(array=w219, new element="c 7", index (row)=6 ("index")) -> (w217:dbl[][])  [unwired: 1 in]
            n148 = Bundle By Name(cluster=w220, "Data Acquisition.Thermistor.Calibration.c"=w217) -> (w221:T2)
          }
          event "c 8": Value Change {
            n149 = event-data() -> ()  [unwired: 1 in, 1 out]
            n150 = Unbundle By Name(w226) -> ("Data Acquisition.Thermistor.Calibration.c"=w225:dbl[][])
            n151 = Replace Array Subset(array=w225, new element="c 8", index (row)=7 ("index")) -> (w223:dbl[][])  [unwired: 1 in]
            n152 = Bundle By Name(cluster=w226, "Data Acquisition.Thermistor.Calibration.c"=w223) -> (w227:T2)
          }
          event "Active": Value Change {
            n153 = event-data() -> ()  [unwired: 1 in, 1 out]
            n154 = Unbundle By Name(w232) -> ("Data Acquisition.Thermistor.Calibration.State"=w231:bool[])
            n155 = Replace Array Subset(array=w231, new element="Active", index=0) -> (w229:bool[])
            n156 = Bundle By Name(cluster=w232, "Data Acquisition.Thermistor.Calibration.State"=w229) -> (w233:T2)
          }
          event "Active 2": Value Change {
            n157 = event-data() -> ()  [unwired: 1 in, 1 out]
            n158 = Unbundle By Name(w238) -> ("Data Acquisition.Thermistor.Calibration.State"=w237:bool[])
            n159 = Replace Array Subset(array=w237, new element="Active 2", index=1) -> (w235:bool[])
            n160 = Bundle By Name(cluster=w238, "Data Acquisition.Thermistor.Calibration.State"=w235) -> (w239:T2)
          }
          event "Active 3": Value Change {
            n161 = event-data() -> ()  [unwired: 1 in, 1 out]
            n162 = Unbundle By Name(w244) -> ("Data Acquisition.Thermistor.Calibration.State"=w243:bool[])
            n163 = Replace Array Subset(array=w243, new element="Active 3", index=2) -> (w241:bool[])
            n164 = Bundle By Name(cluster=w244, "Data Acquisition.Thermistor.Calibration.State"=w241) -> (w245:T2)
          }
          event "Active 4": Value Change {
            n165 = event-data() -> ()  [unwired: 1 in, 1 out]
            n166 = Unbundle By Name(w250) -> ("Data Acquisition.Thermistor.Calibration.State"=w249:bool[])
            n167 = Replace Array Subset(array=w249, new element="Active 4", index=3) -> (w247:bool[])
            n168 = Bundle By Name(cluster=w250, "Data Acquisition.Thermistor.Calibration.State"=w247) -> (w251:T2)
          }
          event "Active 5": Value Change {
            n169 = event-data() -> ()  [unwired: 1 in, 1 out]
            n170 = Unbundle By Name(w256) -> ("Data Acquisition.Thermistor.Calibration.State"=w255:bool[])
            n171 = Replace Array Subset(array=w255, new element="Active 5", index=4) -> (w253:bool[])
            n172 = Bundle By Name(cluster=w256, "Data Acquisition.Thermistor.Calibration.State"=w253) -> (w257:T2)
          }
          event "Active 6": Value Change {
            n173 = event-data() -> ()  [unwired: 1 in, 1 out]
            n174 = Unbundle By Name(w262) -> ("Data Acquisition.Thermistor.Calibration.State"=w261:bool[])
            n175 = Replace Array Subset(array=w261, new element="Active 6", index=5) -> (w259:bool[])
            n176 = Bundle By Name(cluster=w262, "Data Acquisition.Thermistor.Calibration.State"=w259) -> (w263:T2)
          }
          event "Active 7": Value Change {
            n177 = event-data() -> ()  [unwired: 1 in, 1 out]
            n178 = Unbundle By Name(w268) -> ("Data Acquisition.Thermistor.Calibration.State"=w267:bool[])
            n179 = Replace Array Subset(array=w267, new element="Active 7", index=6) -> (w265:bool[])
            n180 = Bundle By Name(cluster=w268, "Data Acquisition.Thermistor.Calibration.State"=w265) -> (w269:T2)
          }
          event "Active 8": Value Change {
            n181 = event-data() -> ()  [unwired: 1 in, 1 out]
            n182 = Unbundle By Name(w274) -> ("Data Acquisition.Thermistor.Calibration.State"=w273:bool[])
            n183 = Replace Array Subset(array=w273, new element="Active 8", index=7) -> (w271:bool[])
            n184 = Bundle By Name(cluster=w274, "Data Acquisition.Thermistor.Calibration.State"=w271) -> (w275:T2)
          }
        }
      }
      "DataCluster out" <- w49
      "State Out" <- w48
    }
  }
